vi "3.5 Downsample.vi"(2 "Corresponding Input Array For Minimum":sgl[](array[numeric]), 3 "Minimum?":bool, 4 "Numeric":i32=91, 5 "Input Array":sgl[](array[numeric])) -> (0 "Corresponding Output Array only for Minimum":sgl[](array[numeric]), 1 "Output Array":sgl[](array[numeric]))   [LabVIEW 2011]
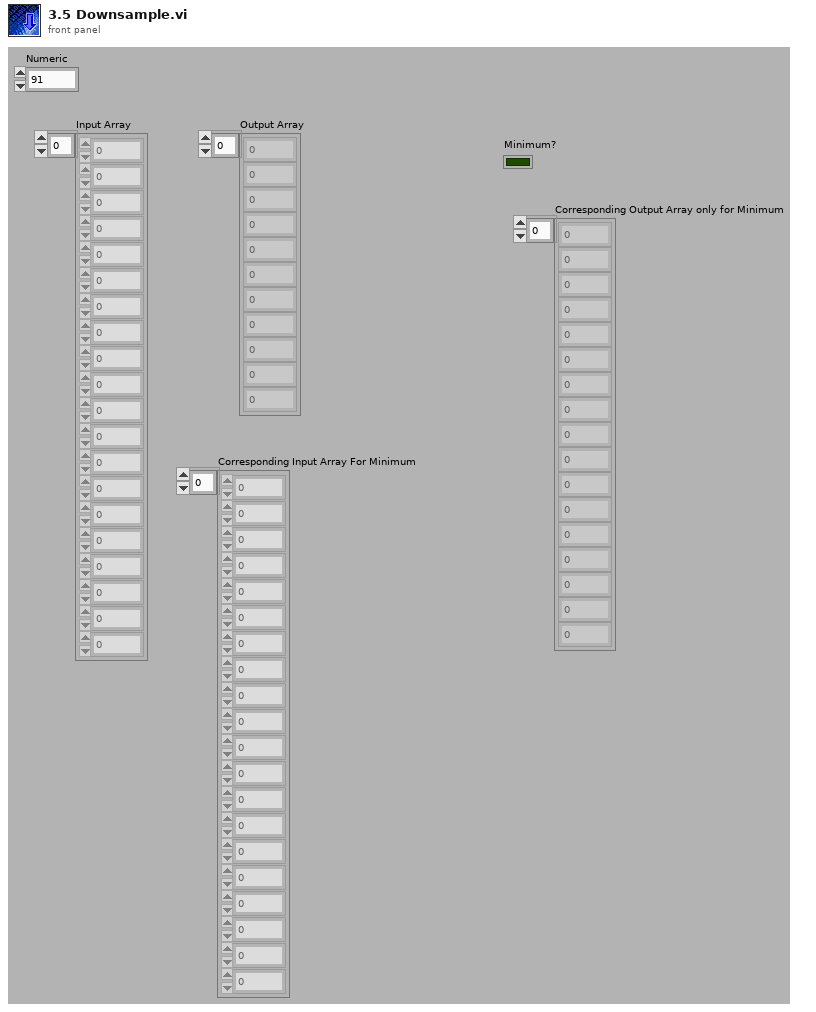
[diagram p1: front panel]
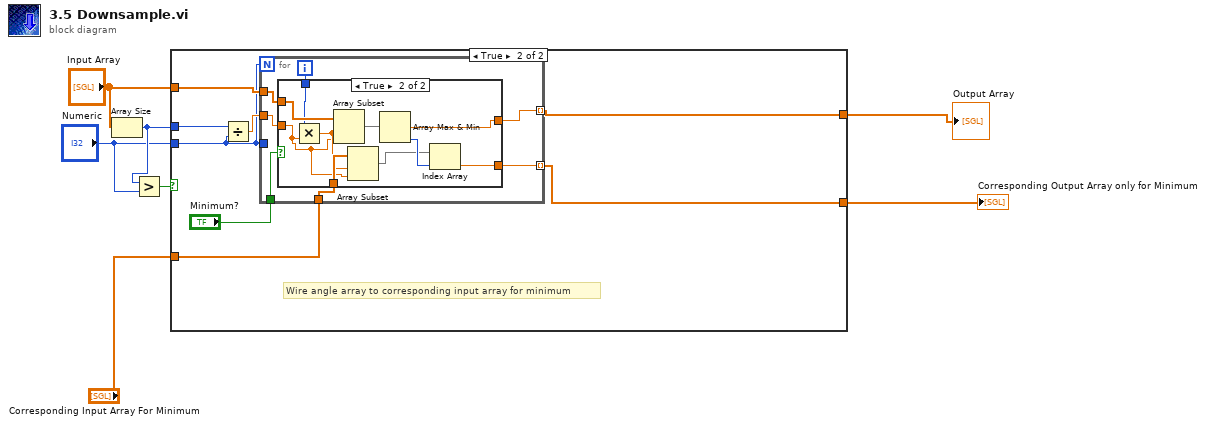
[diagram p0: block diagram]
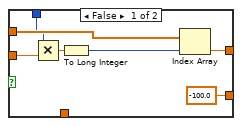
[diagram p3: hidden frame]
diagram:
  n1 = Array Size(array="Input Array") -> (size(s)=w2:i32)
  n2 = Greater?(x=w2, y="Numeric") -> (0:w6:bool)
  n3 = case shown="True" w6 {
    tunnel: w2 -> [_ w17]
    tunnel: "Input Array" -> [w9 w15]
    tunnel: "Numeric" -> [_ w13]
    tunnel: [w9 w12] -> w5
    tunnel: "Corresponding Input Array For Minimum" -> [w8 w11]
    tunnel: [w8 w10] -> w3
    frame False {
    }
    frame True {
      # "Wire angle array to corresponding input array for minimum"
      n4 = Divide(x=w17, y=w13) -> (x/y=w16:dbl)
      n5 = for {
        N: w13 -> [_]
        tunnel: w15 -> [w24]
        tunnel: w16 -> [w22]
        tunnel: [w21] -> w12 mode=indexing
        tunnel: "Minimum?" -> [w20]
        tunnel: w13 -> [_]
        tunnel: w11 -> [w19]
        tunnel: [w18] -> w10 mode=indexing
        i -> [w23]
        n6 = case shown="True" w20 {
          tunnel: w24 -> [w31 w41]
          tunnel: w23 -> [w30 w40]
          tunnel: w22 -> [w28 w32]
          tunnel: [w26 w38] -> w21
          tunnel: w19 -> [_ w35]
          tunnel: [sgl -100.0 ("f") w36] -> w18
          frame False {
            n7 = Multiply(x=w30, y=w28) -> (x*y=w29:dbl)
            n8 = To Long Integer(number=w29) -> (32bit integer=w27:i32)
            n9 = Index Array(array=w31, index=w27) -> (element=w26:sgl)
          }
          frame True {
            n10 = Multiply(x=w40, y=w32) -> (x*y=w33:dbl)
            n11 = Array Subset(array=w41, index=w33, length=w32) -> (w39:sgl[])
            n12 = Array Subset(array=w35, index=w33, length=w32) -> (w34:sgl[])
            n13 = Array Max & Min(array=w39) -> (min value=w38:sgl, min index (indices)=w37:i32)  [unwired: 2 out]
            n14 = Index Array(array=w34, index=w37) -> (element=w36:sgl)
          }
        }
      }
    }
  }
  "Output Array" <- w5
  "Corresponding Output Array only for Minimum" <- w3
